vi "Post Process Files in MultiRun.vi"(3 "Mode":T5=enum."Run VI", 5 "Traverse line In":T2 {"Carrier_2 Q (l/min)" format="%#.2f"; "Row Duration (mins)" format="%#.1f"; "Row No" min=0; "Trace Gas Concentration (%)" min=0.0 format="%#_4f"; "Carrier_1 Q (l/min)" format="%#.4f"; "Tunnel Speed" format="%#.2f"; "Start X" format="%#.2f"; "Start Y" format="%#.2f"; "Start Z" format="%#.2f"; "End X" format="%#.2f"; "End Y" format="%#.2f"; "End Z" format="%#.2f"; "Averaging time (min)" min=0.0 format="%#.2f"}) -> (0 "Error Message":string, 1 "Status":T1, 2 "Traverse line Out":T2 {"Carrier_2 Q (l/min)" format="%#.2f"; "Row Duration (mins)" format="%#.1f"; "Row No" min=0; "Trace Gas Concentration (%)" min=0.0 format="%#_4f"; "Carrier_1 Q (l/min)" format="%#.4f"; "Tunnel Speed" format="%#.2f"; "Start X" format="%#.2f"; "Start Y" format="%#.2f"; "Start Z" format="%#.2f"; "End X" format="%#.2f"; "End Y" format="%#.2f"; "End Z" format="%#.2f"; "Averaging time (min)" min=0.0 format="%#.2f"})   [LabVIEW 2018]
uses:
  Gen Trav/Traverse_cluster.ctl
  Gen Trav/Spacing.ctl
  Controls/Multi_run_mode.ctl
  Controls/User_Specific_mode.ctl
  Gen Trav/Multi_Run_Status.ctl
  Controls/Post_Process.ctl
  Globals/Trav_pos_global.vi
  Globals/Meas_global.vi
panel:
  # "X           Y            Z"
  # "Start"
  # "End"
  # "X           Y            Z"
  # "Start"
  # "End"
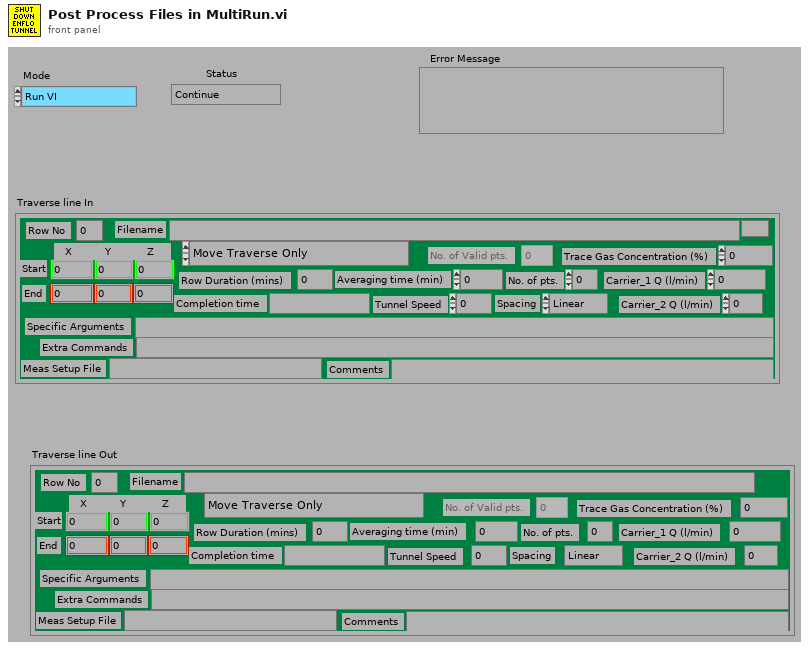
[diagram p1: front panel]
types:
  T1 = typedef "Multi_Run_Status.ctl" = enum16{"Continue", "Continue with Error", "Jump to Next Point", "Jump to Next Row", "Jump To Fall Back", "Terminate Run"}
  T2 = typedef "Traverse_cluster.ctl" = cluster{"Start X":sgl, "Start Y":sgl, "Start Z":sgl, "End X":sgl, "End Y":sgl, "End Z":sgl, "No. of pts.":i32, "Spacing":T3, "Filename":path, "Tunnel Speed":dbl, "Averaging time (min)":dbl, "Extra Commands":string, "Carrier_1 Q (l/min)":dbl, "Carrier_2 Q (l/min)":dbl, "Trace Gas Concentration (%)":dbl, "Specific Arguments":string, "Comments":string, "Row No":i32, "Row Type Selector":T4, "Completion time":string, "Row Duration (mins)":dbl, "No. of Valid pts.":i32, "Meas Setup File":string}
  T3 = typedef "Spacing.ctl" = enum16{"Linear", "Log", "Gauss", "Specified", "N/A"}
  T4 = typedef "Multi_run_mode.ctl" = enum16{"Move Traverse Only", "Set Tunnel Speed Only", "Set Source Only", "Set Measurement Conditions", "Single Measurement", "Vertical Profile", "Lateral Profile", "Longitudinal Profile", "Multi-Axis Profile", "Explore Volume", "Auto Calibrate", "Meas Fast FID Bkgnd", "Check Beam Power", "Scanning Valve Measurement", "Run VI Named:", "Set ADAM Ch", "Wait (minutes)", "Send Message", "Synchronize With:", "Fall Back to this Row", "Turn Off Row Repeating", "Traverse 3D Volume", "Blank Row", "Jump to Fall Back Row"}
  T5 = typedef "User_Specific_mode.ctl" = enum16{"Check VI only", "Run VI"}
  T6 = enum16{"Zero or one", "One", "Zero or more", "One or more"}
  T7 = enum16{"A single file", "Original Results Filenames", "Current Results Filenames"}
  T8 = typedef "Post_Process.ctl" = enum16{"Take New Data", "Post Process Raw Data File"}
  T9 = typedef "PP Raw data file cluster.ctl" = cluster{"Raw Data File":path, "Results File":path}
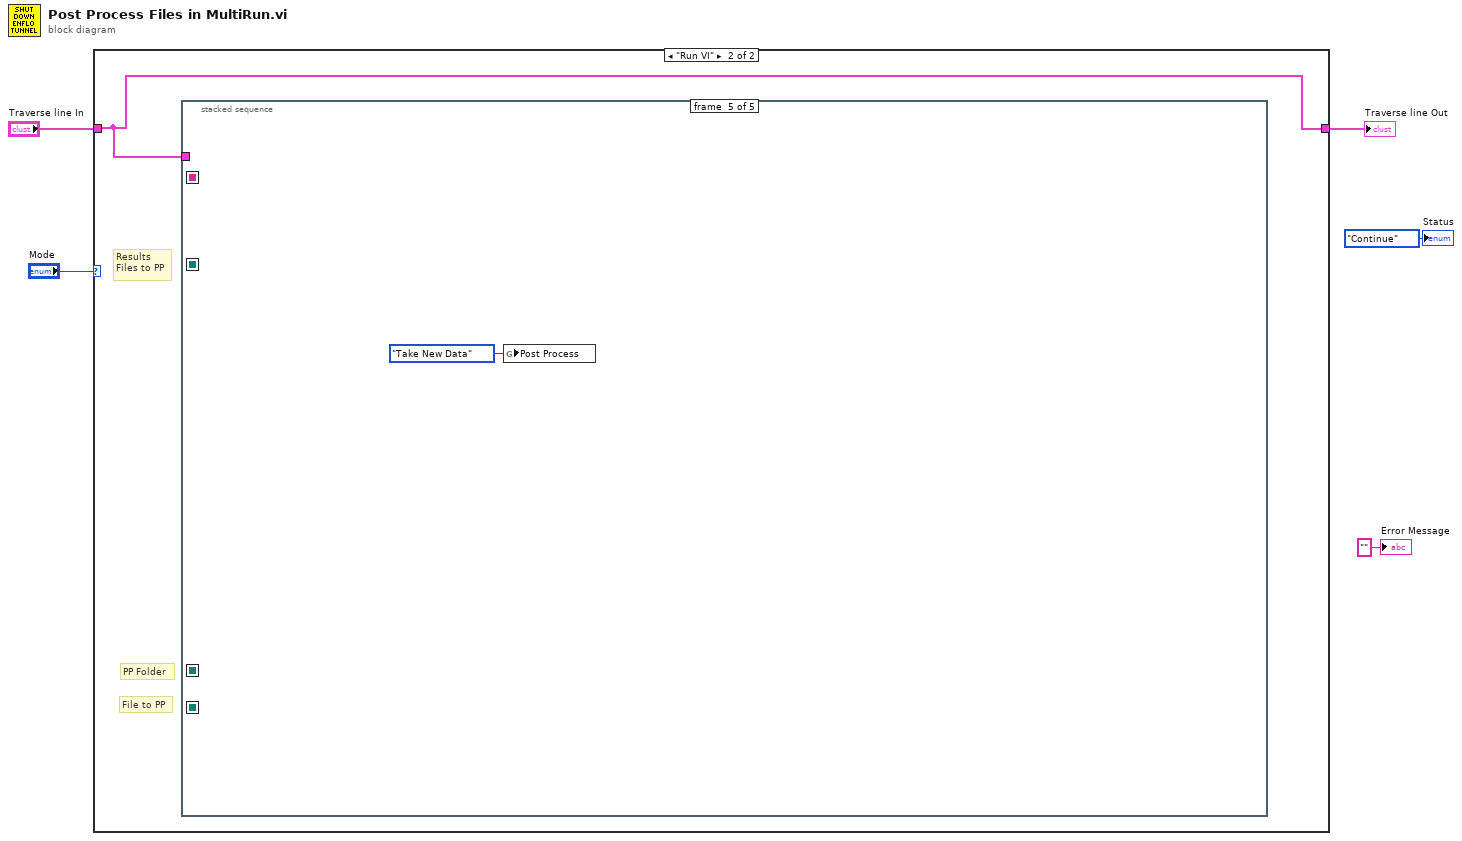
[diagram p0: block diagram]
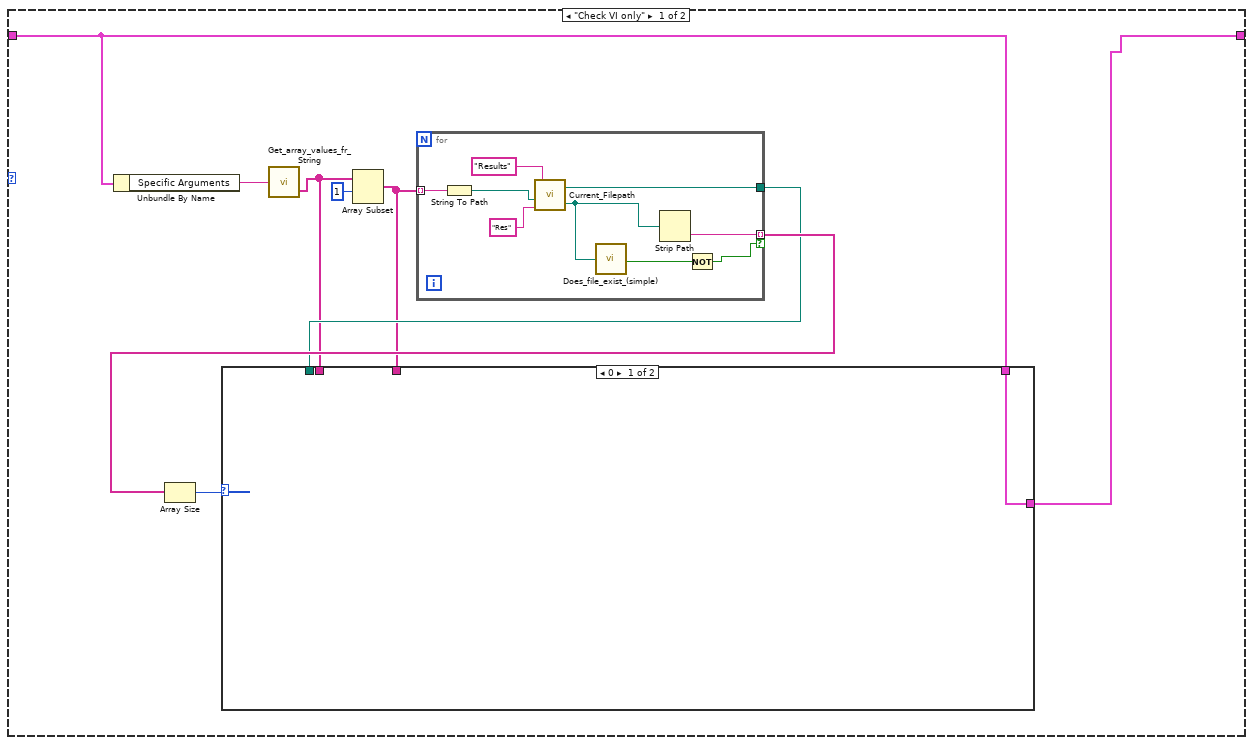
[diagram p2: hidden frame]
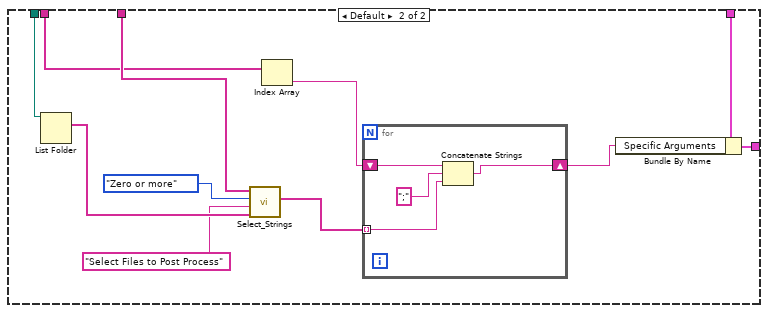
[diagram p3: hidden frame]
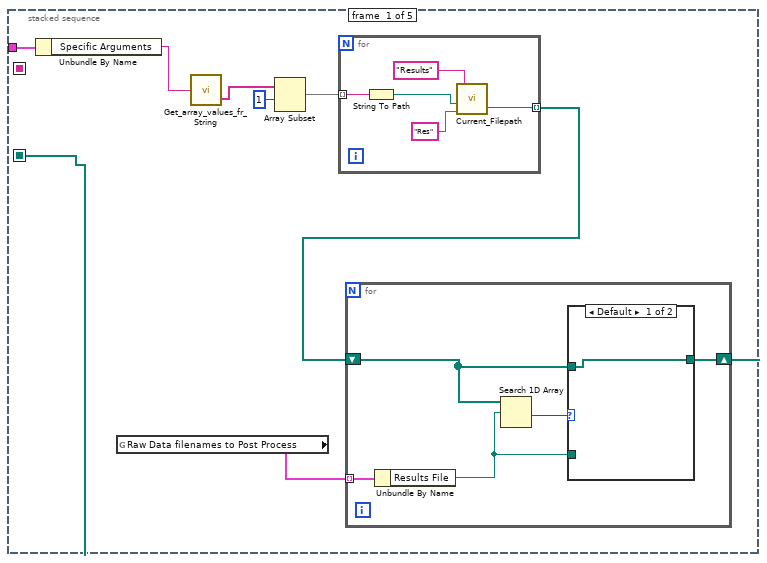
[diagram p4: hidden frame]
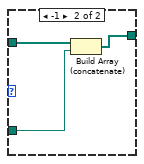
[diagram p5: hidden frame]
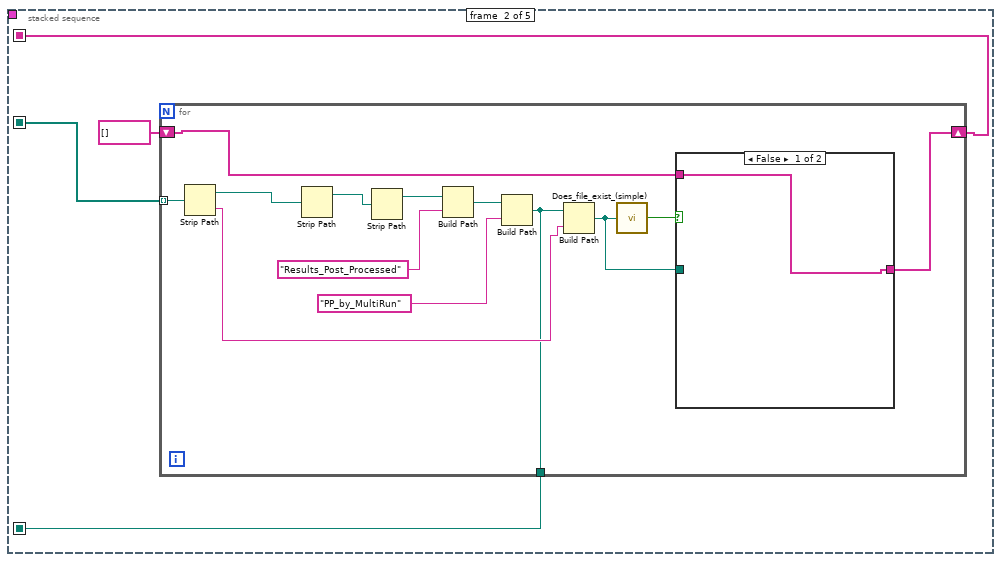
[diagram p6: hidden frame]
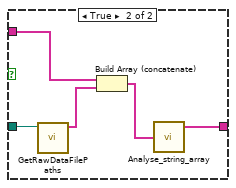
[diagram p7: hidden frame]
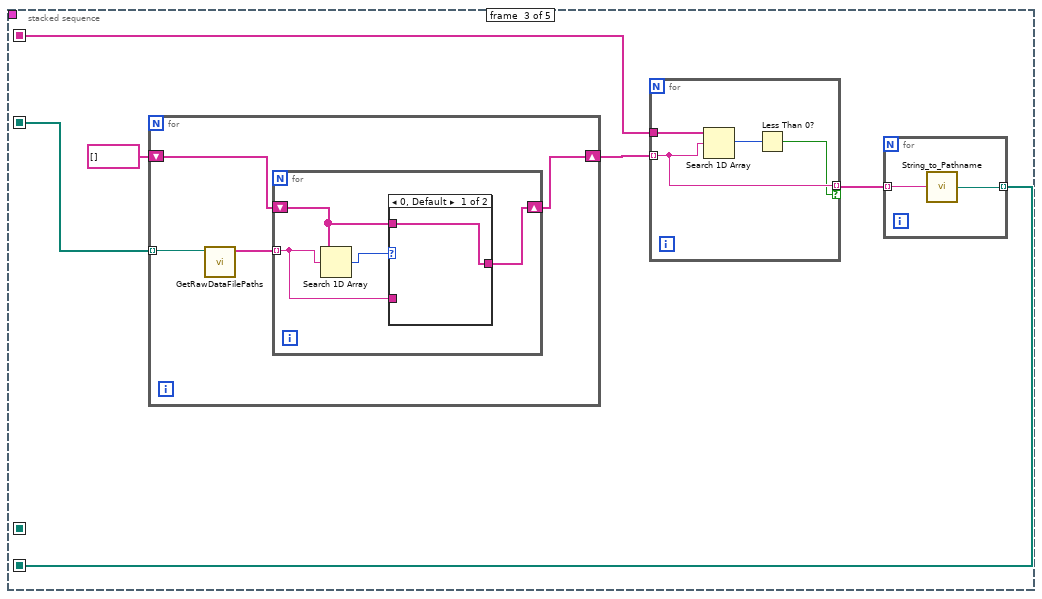
[diagram p8: hidden frame]
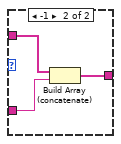
[diagram p9: hidden frame]
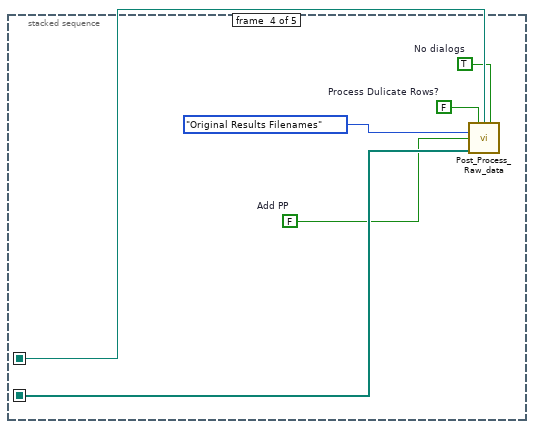
[diagram p10: hidden frame]
diagram:
  n1 = case shown="\"Run VI\"" "Mode" {
    tunnel: "Traverse line In" -> [w7 w40]
    tunnel: [w6 w40] -> w3
    frame "Check VI only" {
      n2 = Unbundle By Name(w7) -> ("Specific Arguments"=w14:string)
      n3 = call "Get_array_values_fr_String.vi"("String Value"=w14) -> ("String array"=w8:string[])  [unwired: 1 out]
      n4 = Array Subset(array=w8, index=1) -> (w9:string[])  [unwired: 1 in]
      n5 = for {
        tunnel: w9 -> [w37] mode=indexing
        tunnel: [w35] -> w10
        tunnel: [w33] -> w12 mode=indexing if=w31
        n6 = String To Path(string=w37) -> (path=w36:path)
        n7 = call "Current_Filepath.vi"("Short_Name"="Res" ("Data Type"), "Filename in"=w36, "Data Type"="Results") -> ("Filename Out"=w34:path, "Directory"=w35:path)  [unwired: 1 in]
        n8 = call "Does_file_exist_(simple).vi"("Pathname"=w34) -> ("exists?"=w32:bool)
        n9 = Strip Path(path=w34) -> (name=w33:string)  [unwired: 1 out]
        n10 = Not(x=w32) -> (.not. x?=w31:bool)
      }
      n11 = Array Size(array=w12) -> (size(s)=w11:i32)
      n12 = case shown="0" w11 {
        tunnel: w10 -> [_ w26]
        tunnel: w9 -> [_ w22]
        tunnel: w8 -> [_ w21]
        tunnel: w7 -> [w15 w18]
        tunnel: [w15 w16] -> w6
        frame 0 {
        }
        frame Default {
          n13 = List Folder(path=w26) -> (filenames=w25:string[])  [unwired: 3 in, 3 out]
          n14 = call "Select_Strings.vi"("Available Ch names"=w25, "Message"="Select Files to Post Process", "Selector mode"=T6."Zero or more", "Desired Ch names (in)"=w22) -> ("Selected Channel Names"=w19:string[])  [unwired: 2 in, 2 out]
          n15 = Index Array(array=w21) -> (element=w20:string)  [unwired: 1 in]
          n16 = for {
            shift-right: [w27] -> w17
            shift-left: w20 -> [w30]
            tunnel: w19 -> [w28] mode=indexing
            n17 = Concatenate Strings(w30, ";" ("string"), w28) -> (w27:string)
          }
          n18 = Bundle By Name(cluster=w18, "Specific Arguments"=w17) -> (w16:T2)
        }
      }
    }
    frame "Run VI" {
      # "File to PP"
      # "PP Folder"
      # "Results\nFiles to PP"
      n19 = stacked-sequence {
        seq-local: [w41 _ _ _ _] -> [_ w66 w91 _ _]
        seq-local: [_ w65 _ _ _] -> [_ _ _ w114 _]
        seq-local: [_ w63 _ _ _] -> [_ _ w89 _ _]
        seq-local: [_ _ w86 _ _] -> [_ _ _ w115 _]
        tunnel: w40 -> [w47 _ _ _ _]
        frame #0 {
          n20 = Unbundle By Name(w47) -> ("Specific Arguments"=w46:string)
          n21 = global read "Trav_pos_global.vi" "Raw Data filenames to Post Process"() -> (w48:T9[])
          n22 = call "Get_array_values_fr_String.vi"("String Value"=w46) -> ("String array"=w45:string[])  [unwired: 1 out]
          n23 = Array Subset(array=w45, index=1) -> (w43:string[])  [unwired: 1 in]
          n24 = for {
            tunnel: w43 -> [w51] mode=indexing
            tunnel: [w49] -> w42 mode=indexing
            n25 = String To Path(string=w51) -> (path=w50:path)
            n26 = call "Current_Filepath.vi"("Short_Name"="Res" ("Data Type"), "Filename in"=w50, "Data Type"="Results") -> ("Filename Out"=w49:path)  [unwired: 1 in, 1 out]
          }
          n27 = for {
            shift-right: [w55] -> w41
            shift-left: w42 -> [w54]
            tunnel: w48 -> [w58] mode=indexing
            n28 = Unbundle By Name(w58) -> ("Results File"=w56:path)
            n29 = Search 1D Array(1D array=w54, element=w56) -> (index of element=w57:i32)  [unwired: 1 in]
            n30 = case shown="Default" w57 {
              tunnel: w56 -> [_ w62]
              tunnel: [w59 w61] -> w55
              tunnel: w54 -> [w59 w60]
              frame Default {
              }
              frame -1 {
                n31 = Build Array (concatenate)(w60, w62) -> (w61:path[])
              }
            }
          }
        }
        frame #1 {
          n32 = for {
            tunnel: w66 -> [w79] mode=indexing
            tunnel: [w71] -> w65
            shift-right: [w67] -> w63
            shift-left: string[] [] ("Unique strings") -> [w68]
            n33 = Strip Path(path=w79) -> (stripped path=w78:path, name=w72:string)
            n34 = Strip Path(path=w78) -> (stripped path=w77:path)  [unwired: 1 out]
            n35 = Strip Path(path=w77) -> (stripped path=w76:path)  [unwired: 1 out]
            n36 = Build Path(base path=w76, name or relative path="Results_Post_Processed") -> (appended path=w73:path)
            n37 = Build Path(base path=w73, name or relative path="PP_by_MultiRun") -> (appended path=w71:path)
            n38 = Build Path(base path=w71, name or relative path=w72) -> (appended path=w69:path)
            n39 = call "Does_file_exist_(simple).vi"("Pathname"=w69) -> ("exists?"=w70:bool)
            n40 = case shown="False" w70 {
              tunnel: w69 -> [_ w85]
              tunnel: w68 -> [w80 w83]
              tunnel: [w80 w81] -> w67
              frame False {
              }
              frame True {
                n41 = call "GetRawDataFilePaths.vi"("Results file or Folder"=w85) -> ("RawDataFilePaths"=w84:string[])  [unwired: 10 in]
                n42 = Build Array (concatenate)(w83, w84) -> (w82:string[])
                n43 = call "Analyse_string_array.vi"("String array"=w82) -> ("Unique strings"=w81:string[])  [unwired: 1 in, 1 out]
              }
            }
          }
        }
        frame #2 {
          n44 = for {
            tunnel: w91 -> [w101] mode=indexing
            shift-right: [w98] -> w88
            shift-left: string[] [] -> [w99]
            n45 = call "GetRawDataFilePaths.vi"("Results file or Folder"=w101) -> ("RawDataFilePaths"=w100:string[])  [unwired: 10 in]
            n46 = for {
              shift-right: [w103] -> w98
              shift-left: w99 -> [w102]
              tunnel: w100 -> [w104] mode=indexing
              n47 = Search 1D Array(1D array=w102, element=w104) -> (index of element=w105:i32)  [unwired: 1 in]
              n48 = case shown="0, Default" w105 {
                tunnel: w104 -> [_ w109]
                tunnel: [w106 w108] -> w103
                tunnel: w102 -> [w106 w107]
                frame 0, Default {
                }
                frame -1 {
                  n49 = Build Array (concatenate)(w107, w109) -> (w108:string[])
                }
              }
            }
          }
          n50 = for {
            tunnel: w89 -> [w95]
            tunnel: w88 -> [w93] mode=indexing
            tunnel: [w93] -> w87 mode=indexing if=w92
            n51 = Search 1D Array(1D array=w95, element=w93) -> (index of element=w94:i32)  [unwired: 1 in]
            n52 = Less Than 0?(x=w94) -> (x < 0?=w92:bool)
          }
          n53 = for {
            tunnel: w87 -> [w97] mode=indexing
            tunnel: [w96] -> w86 mode=indexing
            n54 = call "String_to_Pathname.vi"("Input String"=w97) -> ("path"=w96:path)
          }
        }
        frame #3 {
          w110 = FALSE  # Add PP
          w112 = FALSE  # Process Dulicate Rows?
          w113 = TRUE  # No dialogs
          n55 = call "Post_Process_Raw_data.vi"("Process Dulicate Rows?"=w112, "Post processed Results folder"=w114, "No dialogs"=w113, "Save results to"=T7."Original Results Filenames", "Add PP"=w110, "Selected files"=w115) -> ()  [unwired: 8 in, 2 out]
        }
        frame #4 {
          n56 = global write "Meas_global.vi" "Post Process"(Post_Process."Take New Data" ("Post Process")) -> ()
        }
      }
    }
  }
  "Traverse line Out" <- w3
  "Error Message" <- "" ("Error Message")
  "Status" <- Multi_Run_Status."Continue" ("Status")
